vi "To Variant.vi"(8 "Error In":errorcluster, 11 "TD Flt":refnum<class "Flt.lvclass">) -> (0 "Error Out":errorcluster, 2 "Variant":variant)   [LabVIEW 2020, in "NI_VIAnCFGDataStructure.lvlib" / "Flt.lvclass"]
doc: "Dynamic dispatch interface for conversion of Tree Data classes to variant LV data."
uses:
  <vilib>/addons/analyzer/VIAnCFGDataStructure/Data Types/Float/Flt.lvclass
  <vilib>/addons/analyzer/VIAnCFGDataStructure/Data Types/Float/Flt.lvclass/Flt.ctl
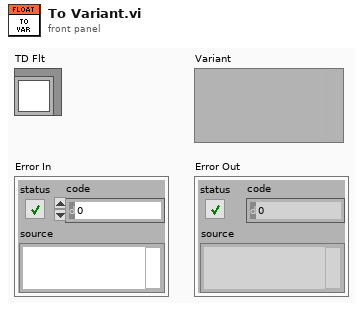
[diagram p1: front panel]
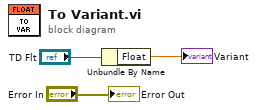
[diagram p0: block diagram]
diagram:
  n1 = Unbundle By Name("TD Flt") -> ("Float"=→"Variant":dbl)
  "Error Out" <- "Error In"
